vi "Upload_photonics_info.vi"() -> ()   [LabVIEW 2017]
panel:
  in  "Upload Wafer to Relations\nTable":bool
  in  "stop":bool
  out "error out":errorcluster
  in  "Upload Detector Mask\nfrom CSV":bool
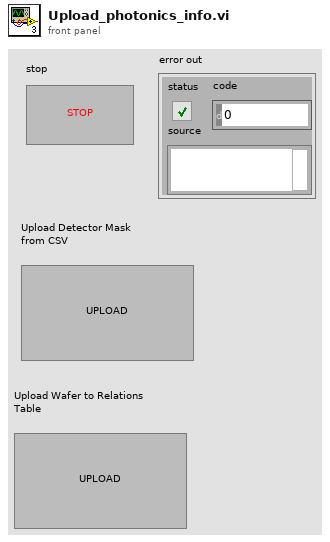
[diagram p1: front panel]
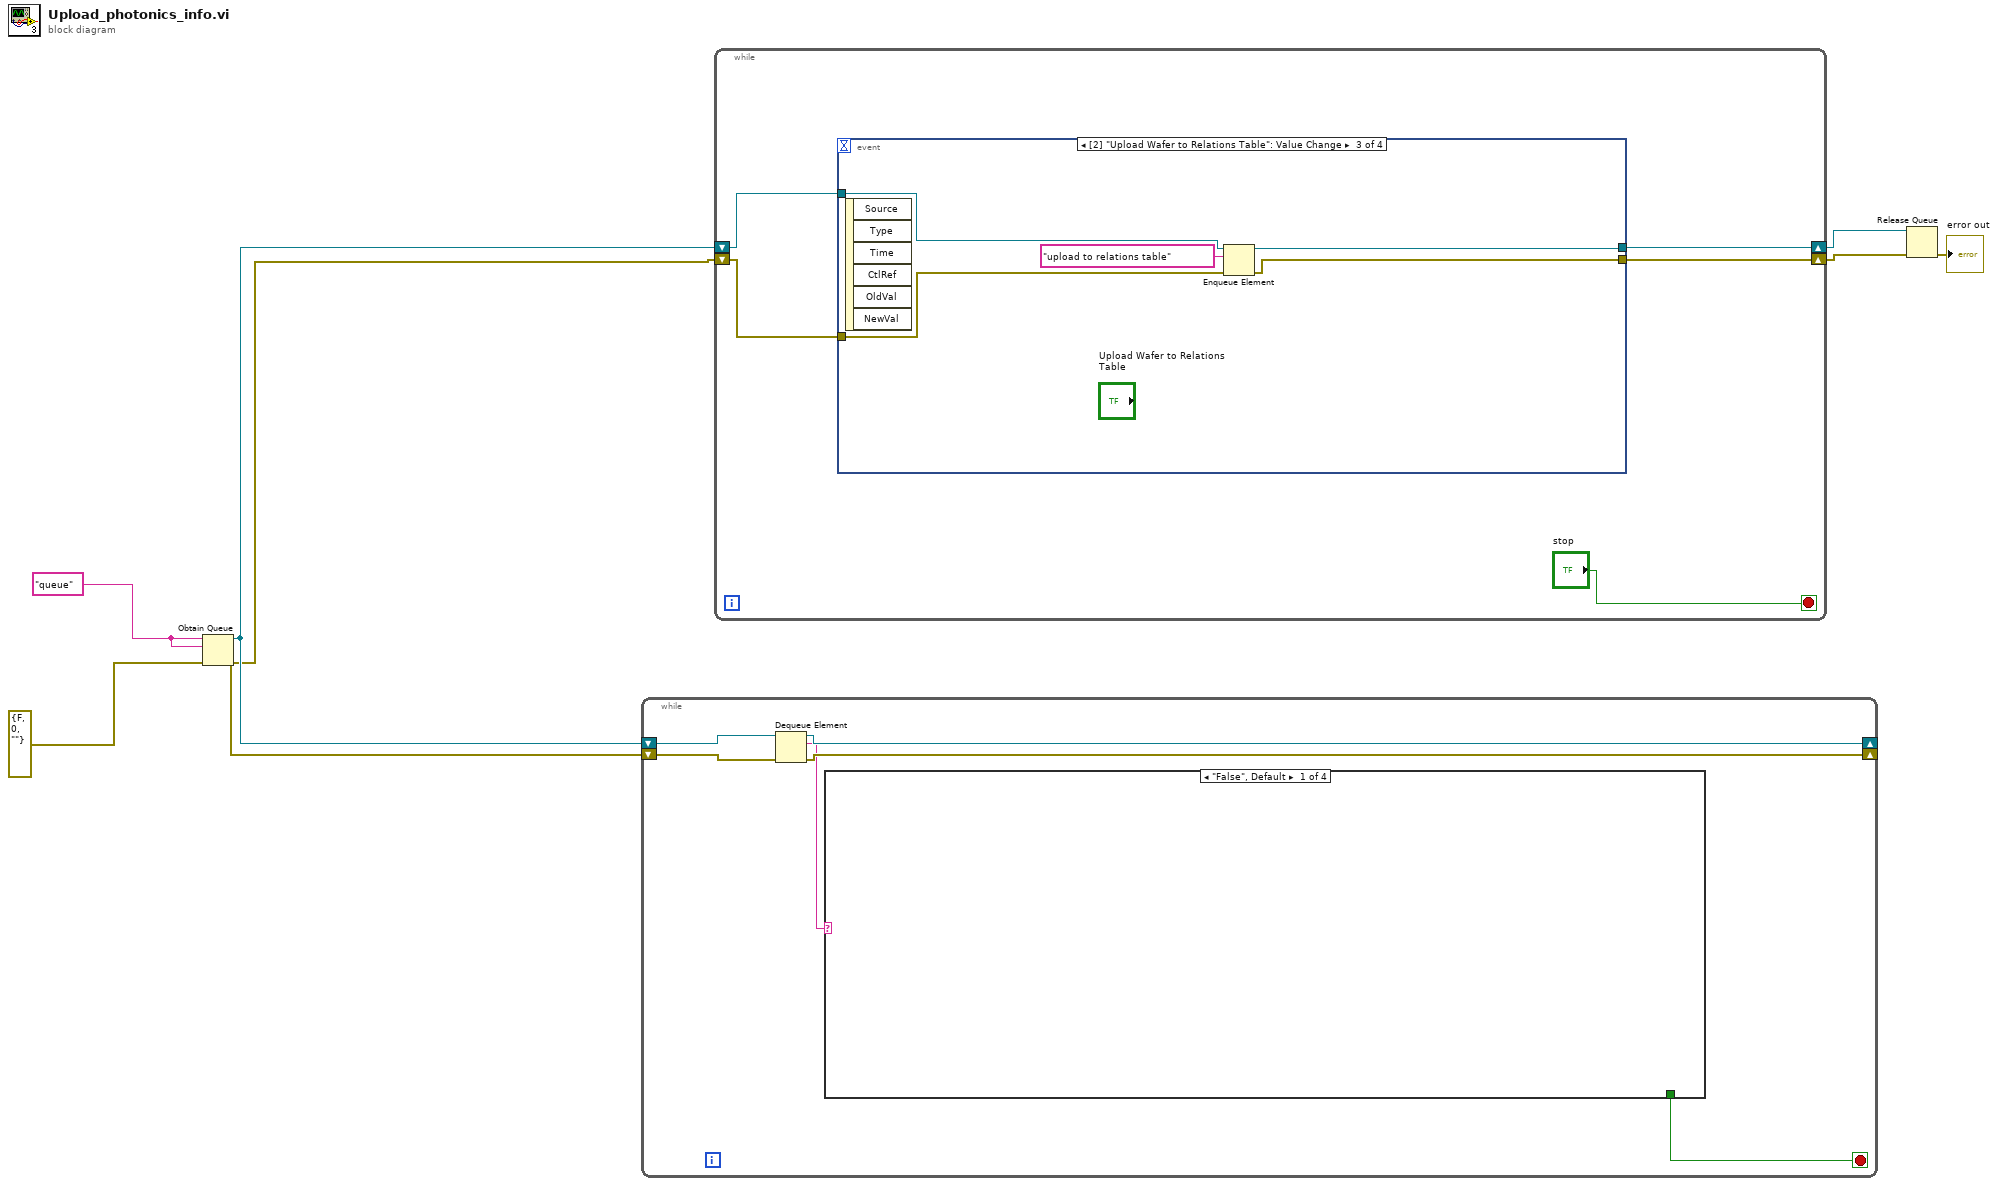
[diagram p0: block diagram]
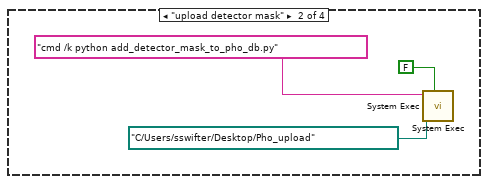
[diagram p2: hidden frame]
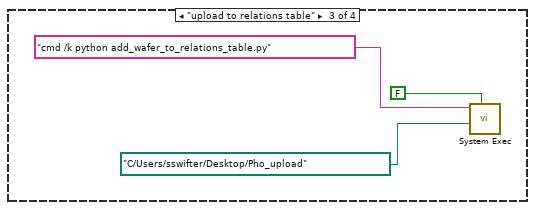
[diagram p3: hidden frame]
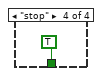
[diagram p4: hidden frame]
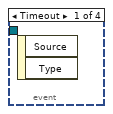
[diagram p5: hidden frame]
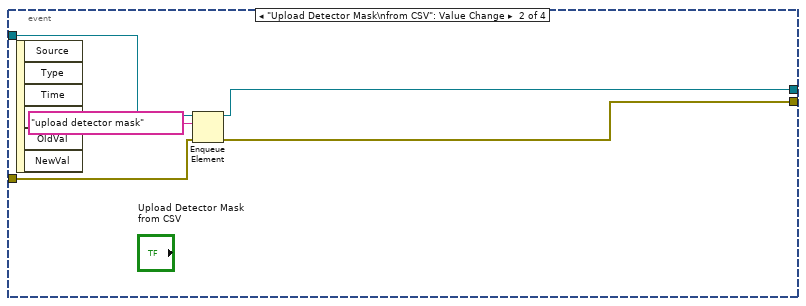
[diagram p6: hidden frame]
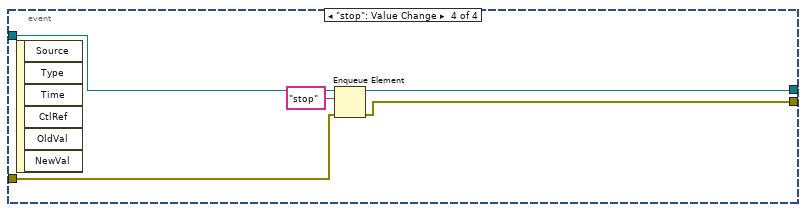
[diagram p7: hidden frame]
diagram:
  w7 = "queue" ("name (unnamed)")
  n1 = Obtain Queue(name (unnamed)=w7, element data type=w7, error in (no error)=errorcluster {"status"=FALSE, "code"=0, "source"=""}) -> (queue out=w5:refnum<queue>, error out=w4:errorcluster)  [unwired: 2 in, 1 out]
  n2 = while {
    shift-right: [w11] -> _
    shift-left: w5 -> [w13]
    shift-right: [w10] -> _
    shift-left: w4 -> [w12]
    stop <- w8 stop-if-true
    n3 = Dequeue Element(queue=w13, error in (no error)=w12) -> (queue out=w11:refnum<queue>, element=w9:string, error out=w10:errorcluster)  [unwired: 1 in, 1 out]
    n4 = case shown="\"False\", Default" w9 {
      tunnel: [_ _ _ TRUE] -> w8
      frame "False", Default {
      }
      frame "upload detector mask" {
        n5 = call <vilib>:"System Exec.vi"("wait until completion? (T)"=FALSE, "working directory"=path "C:/Users/sswifter/Desktop/Pho_upload", "command line"="cmd /k python add_detector_mask_to_pho_db.py") -> ()  [unwired: 5 in, 4 out]
        n6 = call <vilib>:"System Exec.vi"("wait until completion? (T)"=FALSE, "working directory"=path "C:/Users/sswifter/Desktop/Pho_upload", "command line"="cmd /k python add_detector_mask_to_pho_db.py") -> ()  [unwired: 5 in, 4 out]
      }
      frame "upload to relations table" {
        (unwired) FALSE ("wait until completion? (T)")
        n7 = call <vilib>:"System Exec.vi"("wait until completion? (T)"=FALSE, "working directory"=path "C:/Users/sswifter/Desktop/Pho_upload", "command line"="cmd /k python add_wafer_to_relations_table.py") -> ()  [unwired: 5 in, 4 out]
      }
      frame "stop" {
      }
    }
  }
  n8 = while {
    shift-right: [w26] -> w3
    shift-left: w5 -> [w28]
    shift-right: [w25] -> w2
    shift-left: w4 -> [w27]
    stop <- "stop" stop-if-true
    n9 = event shown="[2] \"Upload Wafer to Relations Table\": Value Change" {
      selector: _ -> [_ _ _ _]
      dyn-events: _ -> [_ _ _ _]
      timeout: _ -> [_ _ _ _]
      tunnel: w28 -> [_ w33 w38 w43]
      tunnel: w27 -> [_ w32 w37 w42]
      tunnel: [_ w30 w36 w41] -> w26
      tunnel: [_ w29 w35 w40] -> w25
      event Timeout {
        n10 = event-data() -> ()  [unwired: 1 in, 2 out]
      }
      event "Upload Detector Mask\nfrom CSV": Value Change {
        n11 = event-data() -> ()  [unwired: 1 in, 6 out]
        n12 = Enqueue Element(queue=w33, element="upload detector mask", error in (no error)=w32) -> (queue out=w30:refnum<queue>, error out=w29:errorcluster)  [unwired: 1 in, 1 out]
      }
      event "Upload Wafer to Relations\nTable": Value Change {
        n13 = event-data() -> ()  [unwired: 1 in, 6 out]
        n14 = Enqueue Element(queue=w38, element="upload to relations table", error in (no error)=w37) -> (queue out=w36:refnum<queue>, error out=w35:errorcluster)  [unwired: 1 in, 1 out]
      }
      event "stop": Value Change {
        n15 = event-data() -> ()  [unwired: 1 in, 6 out]
        n16 = Enqueue Element(queue=w43, element="stop", error in (no error)=w42) -> (queue out=w41:refnum<queue>, error out=w40:errorcluster)  [unwired: 1 in, 1 out]
      }
    }
  }
  n17 = Release Queue(queue=w3, error in (no error)=w2) -> (error out=→"error out":errorcluster)  [unwired: 1 in, 2 out]
